vi "Untitled 1 (SubVI).vi"(10 "Y":dbl, 11 "X":dbl) -> (3 "z":dbl)   [LabVIEW 2022 SP3]
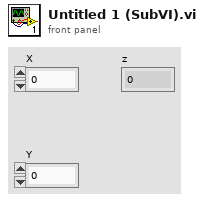
[diagram p1: front panel]
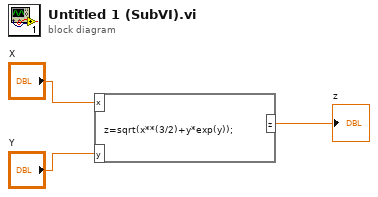
[diagram p0: block diagram]
diagram:
  n1 = formula code="z=sqrt(x**(3/2)+y*exp(y));"("x"="X", "y"="Y") -> ("z"=→"z":dbl)
